vi "IRISS_FPGA_IO_v1.vi"() -> ()   [LabVIEW 2010]
doc: "This VI contains a basic quadrature decoder which is reset asynchronously upon clicking the reset button."
uses:
  <vilib>/platform/TimedLoop/XDataNode/XDataNode.xnode
  <vilib>/Platform/TimedLoop/XDataNode/nitl_modes.ctl
  <vilib>/Platform/TimedLoop/XDataNode/XDNodeRunTimeDep.lvlib
  <vilib>/Platform/TimedLoop/XDataNode/wakeup.ctl
  <vilib>/Platform/TimedLoop/XDataNode/timing_clust.ctl
  <vilib>/eio/EIONode/EIONode.xnode
  Library/KevinLibraryAll/labview/KevLib01.lvlib
  <vilib>/rvi/DataTransferAndStorage/Container/XNode/niFpgaContainer.xnode
  Library/KevinLibraryAll/labview2010/kevLib2010.lvlib
  Library/KevinLibraryAll/labview2010/kevLib2010/FPGA Utilities/Kevins D2A Board/KD2A Port Sel.ctl
panel:
  out "Home L4":bool
  out "Home L1":bool
  out "Home L2":bool
  out "Home L3":bool
  in  "Connector1/DIO19":bool
  in  "Connector1/DIO18":bool
  in  "Connector1/DIO17":bool
  in  "Connector1/DIO16":bool
  in  "Connector1/DIO15":bool
  in  "Connector1/DIO20":bool
  in  "Positive Direction C1-5":bool
  out "JumpBy2Error C1-5":i16
  out "32 bit Position C1-5":i32
  in  "Reset C1-5":bool
  in  "Positive Direction C1-4":bool
  out "JumpBy2Error C1-4":i16
  out "32 bit Position C1-4":i32
  in  "Reset C1-4":bool
  in  "Positive Direction C1-3":bool
  out "JumpBy2Error C1-3":i16
  out "32 bit Position C1-3":i32
  in  "Reset C1-3":bool
  in  "Positive Direction C1-2":bool
  out "JumpBy2Error C1-2":i16
  out "32 bit Position C1-2":i32
  in  "Reset C1-2":bool
  in  "Positive Direction C1-1":bool
  out "JumpBy2Error C1-1":i16
  out "32 bit Position C1-1":i32
  in  "Reset C1-1":bool
  in  "Timeout":i32=40000000
  out "32 bit Position 17":i32
  in  "Reset 17":bool
  in  "Positive Direction 17":bool
  out "JumpBy2Error 17":i16
  out "32 bit Position 16":i32
  in  "Reset 16":bool
  in  "Positive Direction 16":bool
  out "JumpBy2Error 16":i16
  out "32 bit Position 15":i32
  in  "Reset 15":bool
  in  "Positive Direction 15":bool
  out "JumpBy2Error 15":i16
  out "32 bit Position 14":i32
  in  "Reset 14":bool
  in  "Positive Direction 14":bool
  out "JumpBy2Error 14":i16
  out "32 bit Position 13":i32
  in  "Reset 13":bool
  in  "Positive Direction 13":bool
  out "JumpBy2Error 13":i16
  out "32 bit Position 12":i32
  in  "Reset 12":bool
  in  "Positive Direction 12":bool
  out "JumpBy2Error 12":i16
  out "32 bit Position 11":i32
  in  "Reset 11":bool
  in  "Positive Direction 11":bool
  out "JumpBy2Error 11":i16
  out "32 bit Position 10":i32
  in  "Reset 10":bool
  in  "Positive Direction 10":bool
  out "JumpBy2Error 10":i16
  out "32 bit Position 9":i32
  in  "Reset 9":bool
  in  "Positive Direction 9":bool
  out "JumpBy2Error 9":i16
  in  "Positive Direction 8":bool
  out "JumpBy2Error 8":i16
  in  "Positive Direction 7":bool
  out "JumpBy2Error 7":i16
  in  "Positive Direction 6":bool
  out "JumpBy2Error 6":i16
  in  "Reset 5":bool
  in  "Positive Direction 5":bool
  out "JumpBy2Error 5":i16
  out "JumpBy2Error 4":i16
  in  "Positive Direction 4":bool
  out "JumpBy2Error 3":i16
  in  "Positive Direction 3":bool
  out "JumpBy2Error 2":i16
  in  "Positive Direction 2":bool
  out "JumpBy2Error 1":i16
  in  "Positive Direction 1":bool
  out "AI":i16[](array[numeric])
  out "32 bit Position 8":i32
  in  "Reset 8":bool
  out "32 bit Position 7":i32
  in  "Reset 7":bool
  out "32 bit Position 6":i32
  in  "Reset 6":bool
  out "32 bit Position 5":i32
  out "32 bit Position 4":i32
  in  "Reset 4":bool
  out "32 bit Position 3":i32
  in  "Reset 3":bool
  out "32 bit Position 2":i32
  in  "Reset 2":bool
  in  "AO":i16[](array[numeric])=[0, 0, 0, 0, 0, 0, 0, 0]
  out "32 bit Position 1":i32
  in  "Reset 1":bool
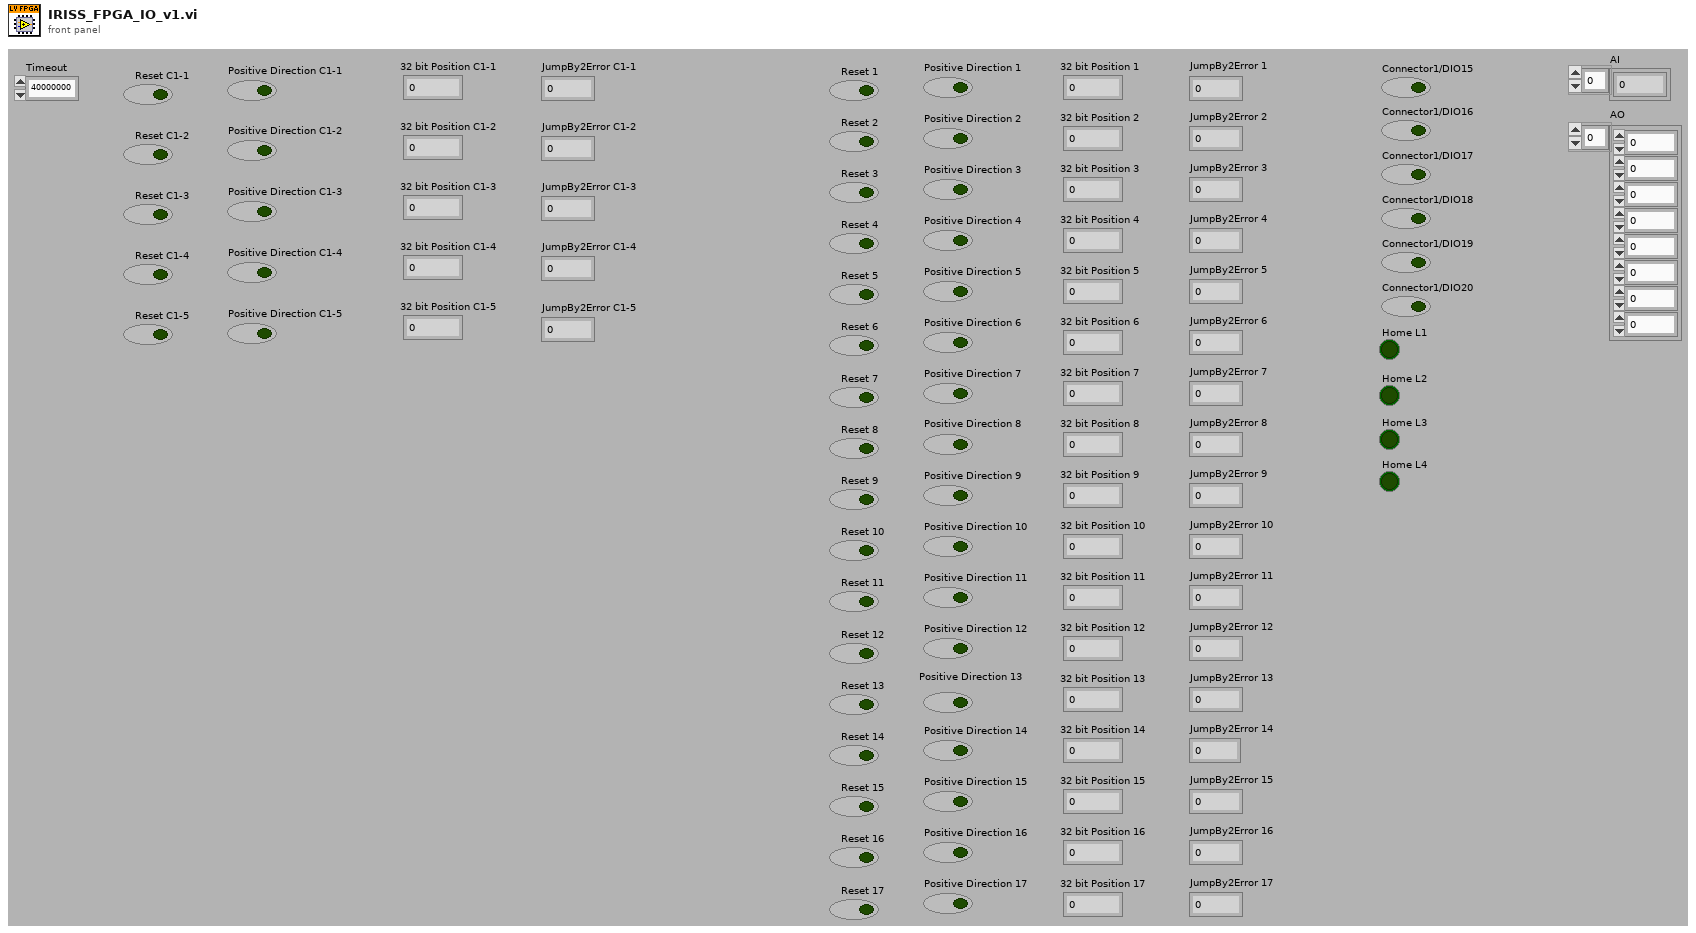
[diagram p1: front panel]
types:
  T1 = typedef "kevLib2010.lvlib/KD2A Port Sel.ctl" = cluster{"Controller Port CLK":refnum<k21>, "Controller Port SIG":refnum<k21>, "DA Port CLK":refnum<k21>, "DA Port SIG":refnum<k21>}
  T2 = typedef "XDNodeRunTimeDep.lvlib/timing_clust.ctl" = cluster{"Expected End [f-1]":u64, "Actual End [f-1]":u64, "Finished Late? [f-1]":bool, "Expected End [i-1]":u64, "Actual End [i-1]":u64, "Finished Late? [i-1]":bool, "Expected Start [i]":u64, "Actual Start [i]":u64, "Expected Start [f]":u64, "Actual Start [f]":u64, "Source Name":string, "Structure Name":string, "Period":i64, "Deadline":i64, "Offset":i64, "Start":i64, "Priority":i32, "Timeout":i32, "Mode":T3, "Wakeup Reason":T4, "Error":errorcluster, "Source Type":string, "Secondary Source Type":string, "Global End Time":u64, "Global Start Time":u64, "Frame Duration":u64, "Iteration Duration":u64, "Assigned CPU":i32, "I/O Scan Engine Mode":u32}
  T3 = typedef "XDNodeRunTimeDep.lvlib/nitl_modes.ctl" = enum32{"No Change", "Process missed periods, maintain original phase", "Discard missed periods, maintain original phase", "Process missed periods, ignore original phase", "Discard missed periods, ignore original phase"}
  T4 = typedef "XDNodeRunTimeDep.lvlib/wakeup.ctl" = enum32{"Normal", "Aborted", "Asynchronous wakeup", "Timing source error", "Timed loop error", "Timeout"}
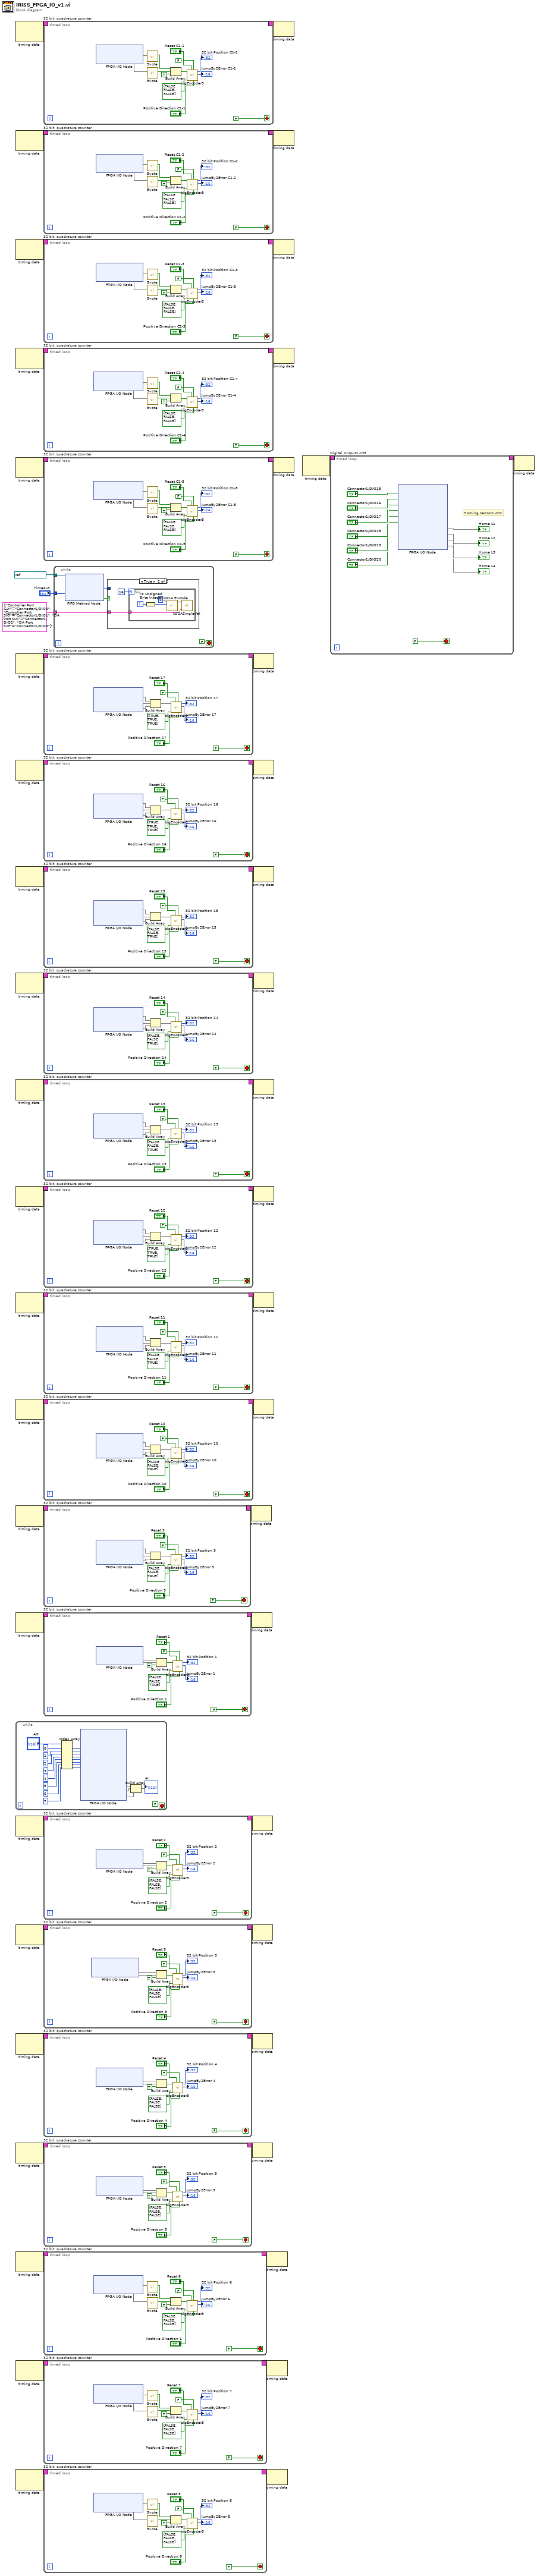
[diagram p0: block diagram]
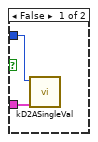
[diagram p2: hidden frame]
diagram:
  n1 = node-c288() -> (w14:T2)  [unwired: 2 out]
  n2 = node-c288() -> (w12:T2)  [unwired: 2 out]
  n3 = node-c288() -> (w10:T2)  [unwired: 2 out]
  n4 = node-c288() -> (w8:T2)  [unwired: 2 out]
  n5 = node-c288() -> (w6:T2)  [unwired: 2 out]
  n6 = node-c288() -> (w17:T2)  [unwired: 2 out]
  n7 = node-c288() -> (w19:T2)  [unwired: 2 out]
  n8 = node-c288() -> (w21:T2)  [unwired: 2 out]
  n9 = node-c288() -> (w23:T2)  [unwired: 2 out]
  n10 = node-c288() -> (w25:T2)  [unwired: 2 out]
  n11 = node-c288() -> (w27:T2)  [unwired: 2 out]
  n12 = node-c288() -> (w29:T2)  [unwired: 2 out]
  n13 = node-c288() -> (w31:T2)  [unwired: 2 out]
  n14 = node-c288() -> (w33:T2)  [unwired: 2 out]
  n15 = node-c288() -> (w48:T2)  [unwired: 2 out]
  n16 = while {
    stop <- FALSE stop-if-true
    n17 = Index Array(array="AO", index #1=0 ("index"), index #2=1 ("index"), index #3=2 ("index"), index #4=3 ("index"), index #5=4 ("index"), index #6=5 ("index"), index #7=6 ("index"), index #8=7 ("index")) -> (element #1=w62:i16, element #2=w61:i16, element #3=w60:i16, element #4=w59:i16, element #5=w58:i16, element #6=w57:i16, element #7=w56:i16, element #8=w55:i16)
    n18 = xnode "FPGA I/O Node"("Connector0/AO0"=w62, "Connector0/AO1"=w61, "Connector0/AO2"=w60, "Connector0/AO3"=w59, "Connector0/AO4"=w58, "Connector0/AO5"=w57, "Connector0/AO6"=w56, "Connector0/AO7"=w55) -> ("Connector0/AI0"=w53, "Connector0/AI1"=w52, "Connector0/AI2"=w50)  [unwired: 11 in, 11 out]
    n19 = Build Array(w53, w52, w50) -> (→"AI":void[])
  }
  n20 = node-c288() -> (w47:T2)  [unwired: 2 out]
  n21 = node-c288() -> (w45:T2)  [unwired: 2 out]
  n22 = node-c288() -> (w43:T2)  [unwired: 2 out]
  n23 = node-c288() -> (w41:T2)  [unwired: 2 out]
  n24 = node-c288() -> (w39:T2)  [unwired: 2 out]
  n25 = node-c288() -> (w37:T2)  [unwired: 2 out]
  n26 = node-c288() -> (w35:T2)  [unwired: 2 out]
  n27 = timed-loop "32 bit, quadrature counter" {
    timing-out: [_] -> w13
    timing: w14 -> [_]
    stop <- FALSE stop-if-true
    n28 = xnode "FPGA I/O Node"() -> ("Connector1/DIO4"=w75, "Connector1/DIO5"=w74)  [unwired: 2 in, 2 out]
    n29 = call "5vote.vi"("Input"=w75) -> ("vote5"=w72:bool)  [unwired: 10 in]
    n30 = call "5vote.vi"("Input"=w74) -> ("vote5"=w73:bool)  [unwired: 10 in]
    n31 = Build Array(w72, w73, TRUE ("element")) -> (w83:bool[])
    n32 = call "bigEncoder3.vi"("Positive Direction"="Positive Direction C1-1", "ForceReset"="Reset C1-1", "Allow C Reset?"=FALSE, "Reset Array"=bool[] [FALSE, FALSE, FALSE], "Encoder Array"=w83) -> ("JumpBy2Error"=→"JumpBy2Error C1-1":i16, "Position"=→"32 bit Position C1-1":i32)  [unwired: 5 out]
  }
  n33 = timed-loop "32 bit, quadrature counter" {
    timing-out: [_] -> w11
    timing: w12 -> [_]
    stop <- FALSE stop-if-true
    n34 = xnode "FPGA I/O Node"() -> ("Connector1/DIO6"=w90, "Connector1/DIO7"=w89)  [unwired: 2 in, 2 out]
    n35 = call "5vote.vi"("Input"=w90) -> ("vote5"=w87:bool)  [unwired: 10 in]
    n36 = call "5vote.vi"("Input"=w89) -> ("vote5"=w88:bool)  [unwired: 10 in]
    n37 = Build Array(w87, w88, TRUE ("element")) -> (w98:bool[])
    n38 = call "bigEncoder3.vi"("Positive Direction"="Positive Direction C1-2", "ForceReset"="Reset C1-2", "Allow C Reset?"=FALSE, "Reset Array"=bool[] [FALSE, FALSE, FALSE], "Encoder Array"=w98) -> ("JumpBy2Error"=→"JumpBy2Error C1-2":i16, "Position"=→"32 bit Position C1-2":i32)  [unwired: 5 out]
  }
  n39 = timed-loop "32 bit, quadrature counter" {
    timing-out: [_] -> w9
    timing: w10 -> [_]
    stop <- FALSE stop-if-true
    n40 = xnode "FPGA I/O Node"() -> ("Connector1/DIO8"=w105, "Connector1/DIO9"=w104)  [unwired: 2 in, 2 out]
    n41 = call "5vote.vi"("Input"=w105) -> ("vote5"=w102:bool)  [unwired: 10 in]
    n42 = call "5vote.vi"("Input"=w104) -> ("vote5"=w103:bool)  [unwired: 10 in]
    n43 = Build Array(w102, w103, TRUE ("element")) -> (w113:bool[])
    n44 = call "bigEncoder3.vi"("Positive Direction"="Positive Direction C1-3", "ForceReset"="Reset C1-3", "Allow C Reset?"=FALSE, "Reset Array"=bool[] [FALSE, FALSE, FALSE], "Encoder Array"=w113) -> ("JumpBy2Error"=→"JumpBy2Error C1-3":i16, "Position"=→"32 bit Position C1-3":i32)  [unwired: 5 out]
  }
  n45 = timed-loop "32 bit, quadrature counter" {
    timing-out: [_] -> w7
    timing: w8 -> [_]
    stop <- FALSE stop-if-true
    n46 = xnode "FPGA I/O Node"() -> ("Connector1/DIO10"=w120, "Connector1/DIO11"=w119)  [unwired: 2 in, 2 out]
    n47 = call "5vote.vi"("Input"=w120) -> ("vote5"=w117:bool)  [unwired: 10 in]
    n48 = call "5vote.vi"("Input"=w119) -> ("vote5"=w118:bool)  [unwired: 10 in]
    n49 = Build Array(w117, w118, TRUE ("element")) -> (w128:bool[])
    n50 = call "bigEncoder3.vi"("Positive Direction"="Positive Direction C1-4", "ForceReset"="Reset C1-4", "Allow C Reset?"=FALSE, "Reset Array"=bool[] [FALSE, FALSE, FALSE], "Encoder Array"=w128) -> ("JumpBy2Error"=→"JumpBy2Error C1-4":i16, "Position"=→"32 bit Position C1-4":i32)  [unwired: 5 out]
  }
  n51 = timed-loop "32 bit, quadrature counter" {
    timing-out: [_] -> w5
    timing: w6 -> [_]
    stop <- FALSE stop-if-true
    n52 = xnode "FPGA I/O Node"() -> ("Connector1/DIO12"=w135, "Connector1/DIO13"=w134)  [unwired: 2 in, 2 out]
    n53 = call "5vote.vi"("Input"=w135) -> ("vote5"=w132:bool)  [unwired: 10 in]
    n54 = call "5vote.vi"("Input"=w134) -> ("vote5"=w133:bool)  [unwired: 10 in]
    n55 = Build Array(w132, w133, TRUE ("element")) -> (w143:bool[])
    n56 = call "bigEncoder3.vi"("Positive Direction"="Positive Direction C1-5", "ForceReset"="Reset C1-5", "Allow C Reset?"=FALSE, "Reset Array"=bool[] [FALSE, FALSE, FALSE], "Encoder Array"=w143) -> ("JumpBy2Error"=→"JumpBy2Error C1-5":i16, "Position"=→"32 bit Position C1-5":i32)  [unwired: 5 out]
  }
  n57 = timed-loop "32 bit, quadrature counter" {
    timing-out: [_] -> w16
    timing: w17 -> [_]
    stop <- FALSE stop-if-true
    n58 = xnode "FPGA I/O Node"() -> ("Connector2/DIO24"=w156, "Connector2/DIO25"=w155, "Connector2/DIO26"=w147)  [unwired: 3 in, 3 out]
    n59 = Build Array(w156, w155, w147) -> (w154:void[])
    n60 = call "bigEncoder3.vi"("Positive Direction"="Positive Direction 17", "ForceReset"="Reset 17", "Allow C Reset?"=FALSE, "Reset Array"=bool[] [TRUE, TRUE, TRUE], "Encoder Array"=w154) -> ("JumpBy2Error"=→"JumpBy2Error 17":i16, "Position"=→"32 bit Position 17":i32)  [unwired: 5 out]
  }
  n61 = timed-loop "32 bit, quadrature counter" {
    timing-out: [_] -> w18
    timing: w19 -> [_]
    stop <- FALSE stop-if-true
    n62 = xnode "FPGA I/O Node"() -> ("Connector2/DIO21"=w169, "Connector2/DIO22"=w168, "Connector2/DIO23"=w160)  [unwired: 3 in, 3 out]
    n63 = Build Array(w169, w168, w160) -> (w167:void[])
    n64 = call "bigEncoder3.vi"("Positive Direction"="Positive Direction 16", "ForceReset"="Reset 16", "Allow C Reset?"=FALSE, "Reset Array"=bool[] [TRUE, TRUE, TRUE], "Encoder Array"=w167) -> ("JumpBy2Error"=→"JumpBy2Error 16":i16, "Position"=→"32 bit Position 16":i32)  [unwired: 5 out]
  }
  n65 = timed-loop "32 bit, quadrature counter" {
    timing-out: [_] -> w20
    timing: w21 -> [_]
    stop <- FALSE stop-if-true
    n66 = xnode "FPGA I/O Node"() -> ("Connector2/DIO18"=w182, "Connector2/DIO19"=w181, "Connector2/DIO20"=w173)  [unwired: 3 in, 3 out]
    n67 = Build Array(w182, w181, w173) -> (w180:void[])
    n68 = call "bigEncoder3.vi"("Positive Direction"="Positive Direction 15", "ForceReset"="Reset 15", "Allow C Reset?"=FALSE, "Reset Array"=bool[] [FALSE, FALSE, TRUE], "Encoder Array"=w180) -> ("JumpBy2Error"=→"JumpBy2Error 15":i16, "Position"=→"32 bit Position 15":i32)  [unwired: 5 out]
  }
  n69 = timed-loop "32 bit, quadrature counter" {
    timing-out: [_] -> w22
    timing: w23 -> [_]
    stop <- FALSE stop-if-true
    n70 = xnode "FPGA I/O Node"() -> ("Connector2/DIO15"=w195, "Connector2/DIO16"=w194, "Connector2/DIO17"=w186)  [unwired: 3 in, 3 out]
    n71 = Build Array(w195, w194, w186) -> (w193:void[])
    n72 = call "bigEncoder3.vi"("Positive Direction"="Positive Direction 14", "ForceReset"="Reset 14", "Allow C Reset?"=FALSE, "Reset Array"=bool[] [FALSE, FALSE, TRUE], "Encoder Array"=w193) -> ("JumpBy2Error"=→"JumpBy2Error 14":i16, "Position"=→"32 bit Position 14":i32)  [unwired: 5 out]
  }
  n73 = timed-loop "32 bit, quadrature counter" {
    timing-out: [_] -> w24
    timing: w25 -> [_]
    stop <- FALSE stop-if-true
    n74 = xnode "FPGA I/O Node"() -> ("Connector2/DIO12"=w208, "Connector2/DIO13"=w207, "Connector2/DIO14"=w199)  [unwired: 3 in, 3 out]
    n75 = Build Array(w208, w207, w199) -> (w206:void[])
    n76 = call "bigEncoder3.vi"("Positive Direction"="Positive Direction 13", "ForceReset"="Reset 13", "Allow C Reset?"=FALSE, "Reset Array"=bool[] [FALSE, FALSE, TRUE], "Encoder Array"=w206) -> ("JumpBy2Error"=→"JumpBy2Error 13":i16, "Position"=→"32 bit Position 13":i32)  [unwired: 5 out]
  }
  n77 = timed-loop "32 bit, quadrature counter" {
    timing-out: [_] -> w26
    timing: w27 -> [_]
    stop <- FALSE stop-if-true
    n78 = xnode "FPGA I/O Node"() -> ("Connector2/DIO9"=w221, "Connector2/DIO10"=w220, "Connector2/DIO11"=w212)  [unwired: 3 in, 3 out]
    n79 = Build Array(w221, w220, w212) -> (w219:void[])
    n80 = call "bigEncoder3.vi"("Positive Direction"="Positive Direction 12", "ForceReset"="Reset 12", "Allow C Reset?"=FALSE, "Reset Array"=bool[] [TRUE, TRUE, TRUE], "Encoder Array"=w219) -> ("JumpBy2Error"=→"JumpBy2Error 12":i16, "Position"=→"32 bit Position 12":i32)  [unwired: 5 out]
  }
  n81 = timed-loop "32 bit, quadrature counter" {
    timing-out: [_] -> w28
    timing: w29 -> [_]
    stop <- FALSE stop-if-true
    n82 = xnode "FPGA I/O Node"() -> ("Connector2/DIO6"=w234, "Connector2/DIO7"=w233, "Connector2/DIO8"=w225)  [unwired: 3 in, 3 out]
    n83 = Build Array(w234, w233, w225) -> (w232:void[])
    n84 = call "bigEncoder3.vi"("Positive Direction"="Positive Direction 11", "ForceReset"="Reset 11", "Allow C Reset?"=FALSE, "Reset Array"=bool[] [FALSE, FALSE, TRUE], "Encoder Array"=w232) -> ("JumpBy2Error"=→"JumpBy2Error 11":i16, "Position"=→"32 bit Position 11":i32)  [unwired: 5 out]
  }
  n85 = timed-loop "32 bit, quadrature counter" {
    timing-out: [_] -> w30
    timing: w31 -> [_]
    stop <- FALSE stop-if-true
    n86 = xnode "FPGA I/O Node"() -> ("Connector2/DIO3"=w247, "Connector2/DIO4"=w246, "Connector2/DIO5"=w238)  [unwired: 3 in, 3 out]
    n87 = Build Array(w247, w246, w238) -> (w245:void[])
    n88 = call "bigEncoder3.vi"("Positive Direction"="Positive Direction 10", "ForceReset"="Reset 10", "Allow C Reset?"=FALSE, "Reset Array"=bool[] [FALSE, FALSE, TRUE], "Encoder Array"=w245) -> ("JumpBy2Error"=→"JumpBy2Error 10":i16, "Position"=→"32 bit Position 10":i32)  [unwired: 5 out]
  }
  n89 = timed-loop "32 bit, quadrature counter" {
    timing-out: [_] -> w32
    timing: w33 -> [_]
    stop <- FALSE stop-if-true
    n90 = xnode "FPGA I/O Node"() -> ("Connector2/DIO0"=w260, "Connector2/DIO1"=w259, "Connector2/DIO2"=w251)  [unwired: 3 in, 3 out]
    n91 = Build Array(w260, w259, w251) -> (w258:void[])
    n92 = call "bigEncoder3.vi"("Positive Direction"="Positive Direction 9", "ForceReset"="Reset 9", "Allow C Reset?"=FALSE, "Reset Array"=bool[] [FALSE, FALSE, TRUE], "Encoder Array"=w258) -> ("JumpBy2Error"=→"JumpBy2Error 9":i16, "Position"=→"32 bit Position 9":i32)  [unwired: 5 out]
  }
  n93 = timed-loop "32 bit, quadrature counter" {
    timing-out: [_] -> w49
    timing: w48 -> [_]
    stop <- FALSE stop-if-true
    n94 = xnode "FPGA I/O Node"() -> ("Connector0/DIO0"=w273, "Connector0/DIO1"=w272)  [unwired: 2 in, 2 out]
    n95 = Build Array(w273, w272, TRUE ("element")) -> (w271:bool[])
    n96 = call "bigEncoder3.vi"("Positive Direction"="Positive Direction 1", "ForceReset"="Reset 1", "Allow C Reset?"=FALSE, "Reset Array"=bool[] [FALSE, FALSE, TRUE], "Encoder Array"=w271) -> ("JumpBy2Error"=→"JumpBy2Error 1":i16, "Position"=→"32 bit Position 1":i32)  [unwired: 5 out]
  }
  n97 = timed-loop "32 bit, quadrature counter" {
    timing-out: [_] -> w46
    timing: w47 -> [_]
    stop <- FALSE stop-if-true
    n98 = xnode "FPGA I/O Node"() -> ("Connector0/DIO2"=w281, "Connector0/DIO3"=w280)  [unwired: 2 in, 2 out]
    n99 = Build Array(w281, w280, TRUE ("element")) -> (w286:bool[])
    n100 = call "bigEncoder3.vi"("Positive Direction"="Positive Direction 2", "ForceReset"="Reset 2", "Allow C Reset?"=FALSE, "Reset Array"=bool[] [FALSE, FALSE, FALSE], "Encoder Array"=w286) -> ("JumpBy2Error"=→"JumpBy2Error 2":i16, "Position"=→"32 bit Position 2":i32)  [unwired: 5 out]
  }
  n101 = timed-loop "32 bit, quadrature counter" {
    timing-out: [_] -> w44
    timing: w45 -> [_]
    stop <- FALSE stop-if-true
    n102 = xnode "FPGA I/O Node"() -> ("Connector0/DIO4"=w293, "Connector0/DIO5"=w292)  [unwired: 2 in, 2 out]
    n103 = Build Array(w293, w292, TRUE ("element")) -> (w299:bool[])
    n104 = call "bigEncoder3.vi"("Positive Direction"="Positive Direction 3", "ForceReset"="Reset 3", "Allow C Reset?"=FALSE, "Reset Array"=bool[] [FALSE, FALSE, FALSE], "Encoder Array"=w299) -> ("JumpBy2Error"=→"JumpBy2Error 3":i16, "Position"=→"32 bit Position 3":i32)  [unwired: 5 out]
  }
  n105 = timed-loop "32 bit, quadrature counter" {
    timing-out: [_] -> w42
    timing: w43 -> [_]
    stop <- FALSE stop-if-true
    n106 = xnode "FPGA I/O Node"() -> ("Connector0/DIO6"=w306, "Connector0/DIO7"=w305)  [unwired: 2 in, 2 out]
    n107 = Build Array(w306, w305, TRUE ("element")) -> (w312:bool[])
    n108 = call "bigEncoder3.vi"("Positive Direction"="Positive Direction 4", "ForceReset"="Reset 4", "Allow C Reset?"=FALSE, "Reset Array"=bool[] [FALSE, FALSE, FALSE], "Encoder Array"=w312) -> ("JumpBy2Error"=→"JumpBy2Error 4":i16, "Position"=→"32 bit Position 4":i32)  [unwired: 5 out]
  }
  n109 = timed-loop "32 bit, quadrature counter" {
    timing-out: [_] -> w40
    timing: w41 -> [_]
    stop <- FALSE stop-if-true
    n110 = xnode "FPGA I/O Node"() -> ("Connector0/DIO8"=w316, "Connector0/DIO9"=w317)  [unwired: 2 in, 2 out]
    n111 = Build Array(w316, w317, TRUE ("element")) -> (w325:bool[])
    n112 = call "bigEncoder3.vi"("Positive Direction"="Positive Direction 5", "ForceReset"="Reset 5", "Allow C Reset?"=FALSE, "Reset Array"=bool[] [FALSE, FALSE, FALSE], "Encoder Array"=w325) -> ("JumpBy2Error"=→"JumpBy2Error 5":i16, "Position"=→"32 bit Position 5":i32)  [unwired: 5 out]
  }
  n113 = timed-loop "32 bit, quadrature counter" {
    timing-out: [_] -> w38
    timing: w39 -> [_]
    stop <- FALSE stop-if-true
    n114 = xnode "FPGA I/O Node"() -> ("Connector0/DIO10"=w332, "Connector0/DIO11"=w331)  [unwired: 2 in, 2 out]
    n115 = call "5vote.vi"("Input"=w332) -> ("vote5"=w329:bool)  [unwired: 10 in]
    n116 = call "5vote.vi"("Input"=w331) -> ("vote5"=w330:bool)  [unwired: 10 in]
    n117 = Build Array(w329, w330, TRUE ("element")) -> (w340:bool[])
    n118 = call "bigEncoder3.vi"("Positive Direction"="Positive Direction 6", "ForceReset"="Reset 6", "Allow C Reset?"=FALSE, "Reset Array"=bool[] [FALSE, FALSE, FALSE], "Encoder Array"=w340) -> ("JumpBy2Error"=→"JumpBy2Error 6":i16, "Position"=→"32 bit Position 6":i32)  [unwired: 5 out]
  }
  n119 = timed-loop "32 bit, quadrature counter" {
    timing-out: [_] -> w36
    timing: w37 -> [_]
    stop <- FALSE stop-if-true
    n120 = xnode "FPGA I/O Node"() -> ("Connector0/DIO12"=w347, "Connector0/DIO13"=w345)  [unwired: 2 in, 2 out]
    n121 = call "5vote.vi"("Input"=w347) -> ("vote5"=w346:bool)  [unwired: 10 in]
    n122 = call "5vote.vi"("Input"=w345) -> ("vote5"=w344:bool)  [unwired: 10 in]
    n123 = Build Array(w346, w344, TRUE ("element")) -> (w355:bool[])
    n124 = call "bigEncoder3.vi"("Positive Direction"="Positive Direction 7", "ForceReset"="Reset 7", "Allow C Reset?"=FALSE, "Reset Array"=bool[] [FALSE, FALSE, FALSE], "Encoder Array"=w355) -> ("JumpBy2Error"=→"JumpBy2Error 7":i16, "Position"=→"32 bit Position 7":i32)  [unwired: 5 out]
  }
  n125 = timed-loop "32 bit, quadrature counter" {
    timing-out: [_] -> w34
    timing: w35 -> [_]
    stop <- FALSE stop-if-true
    n126 = xnode "FPGA I/O Node"() -> ("Connector0/DIO14"=w360, "Connector0/DIO15"=w362)  [unwired: 2 in, 2 out]
    n127 = call "5vote.vi"("Input"=w360) -> ("vote5"=w359:bool)  [unwired: 10 in]
    n128 = call "5vote.vi"("Input"=w362) -> ("vote5"=w361:bool)  [unwired: 10 in]
    n129 = Build Array(w359, w361, TRUE ("element")) -> (w370:bool[])
    n130 = call "bigEncoder3.vi"("Positive Direction"="Positive Direction 8", "ForceReset"="Reset 8", "Allow C Reset?"=FALSE, "Reset Array"=bool[] [FALSE, FALSE, FALSE], "Encoder Array"=w370) -> ("JumpBy2Error"=→"JumpBy2Error 8":i16, "Position"=→"32 bit Position 8":i32)  [unwired: 5 out]
  }
  n131 = while {
    tunnel: refnum<k21> "DA Transfer" ("FIFO Out") -> [w379]
    tunnel: "Timeout" -> [w378]
    tunnel: T1 {"Controller Port CLK"="Connector1/DIO0", "Controller Port SIG"="Connector1/DIO1", "DA Port CLK"="Connector1/DIO2", "DA Port SIG"="Connector1/DIO3"} ("DIO Port Selection") -> [w375]
    stop <- FALSE stop-if-true
    n132 = xnode ("FIFO Method Node")("Timeout"=w378, "FIFO In"=w379) -> ("Element"=w376:u16, "Timed Out?"=w377:bool)  [unwired: 1 out]
    n133 = case shown="True" w377 {
      tunnel: w376 -> [w381 _]
      tunnel: w375 -> [w380 w382]
      frame False {
        n134 = call "kD2ASingleVal.vi"("DIO Port Selection"=w380, "Single Input Element"=w381) -> ()  [unwired: 10 in]
      }
      frame True {
        n135 = for {
          N: 16 -> [_]
          tunnel: w382 -> [w384]
          i -> [w388]
          n136 = To Unsigned Byte Integer(number=w388) -> (unsigned 8bit integer=w387:u8)
          n137 = call "kD2A Encode.vi"("Position"=w387, "Value"=i16 0) -> ("Coded Output"=w385:u16)  [unwired: 9 in]
          n138 = call "kD2ASingleVal.vi"("DIO Port Selection"=w384, "Single Input Element"=w385) -> ()  [unwired: 10 in]
        }
      }
    }
  }
  n139 = node-c288(w32) -> ()  [unwired: 1 out]
  n140 = node-c288(w49) -> ()  [unwired: 1 out]
  n141 = node-c288(w46) -> ()  [unwired: 1 out]
  n142 = node-c288(w44) -> ()  [unwired: 1 out]
  n143 = node-c288(w42) -> ()  [unwired: 1 out]
  n144 = node-c288(w40) -> ()  [unwired: 1 out]
  n145 = node-c288(w16) -> ()  [unwired: 1 out]
  n146 = node-c288(w18) -> ()  [unwired: 1 out]
  n147 = node-c288(w20) -> ()  [unwired: 1 out]
  n148 = node-c288(w22) -> ()  [unwired: 1 out]
  n149 = node-c288(w24) -> ()  [unwired: 1 out]
  n150 = node-c288(w26) -> ()  [unwired: 1 out]
  n151 = node-c288(w28) -> ()  [unwired: 1 out]
  n152 = node-c288(w30) -> ()  [unwired: 1 out]
  n153 = node-c288(w38) -> ()  [unwired: 1 out]
  n154 = node-c288(w36) -> ()  [unwired: 1 out]
  n155 = node-c288(w34) -> ()  [unwired: 1 out]
  n156 = node-c288(w13) -> ()  [unwired: 1 out]
  n157 = node-c288(w11) -> ()  [unwired: 1 out]
  n158 = node-c288(w9) -> ()  [unwired: 1 out]
  n159 = node-c288(w7) -> ()  [unwired: 1 out]
  n160 = node-c288(w5) -> ()  [unwired: 1 out]
  n161 = node-c288() -> (w2:T2)  [unwired: 2 out]
  n162 = timed-loop "Digital Outputs -MG" {
    timing-out: [_] -> w1
    timing: w2 -> [_]
    stop <- FALSE stop-if-true
    # "Homing sensors -CW"
    n163 = xnode "FPGA I/O Node"("Connector1/DIO15"="Connector1/DIO15", "Connector1/DIO16"="Connector1/DIO16", "Connector1/DIO17"="Connector1/DIO17", "Connector1/DIO18"="Connector1/DIO18", "Connector1/DIO19"="Connector1/DIO19", "Connector1/DIO20"="Connector1/DIO20") -> ("Connector1/DIO21"=→"Home L1", "Connector1/DIO22"=→"Home L2", "Connector1/DIO23"=→"Home L3", "Connector1/DIO24"=→"Home L4")  [unwired: 10 in, 10 out]
  }
  n164 = node-c288(w1) -> ()  [unwired: 1 out]
